vi "myBuriedIntelligence.vi"() -> ()   [LabVIEW 2016]
panel:
  in  "Tab Control":enum32{"Page 1"}(tab)
  out "Array 2":bool[][](array[boolean])
  in  "speed":dbl(slide) scale=0.0..10.0
  in  "Stop":bool
  out "Chosen Path":path
  in  "JPG/JEPG":bool
  in  "Choose Pic Path":path
  out "String":string
  in  "Choose Text Path":path
  out "Read Pic":picture
  out "new picture":picture
  in  "Before Embeded":path
  in  "After Embeded":path
  out "ChosenPath":path
  out "String 2":string
  out "String 3":string
  out "Decoded String":string
  out "Decoded Words Size":i32
  out "Array":bool[][](array[boolean])
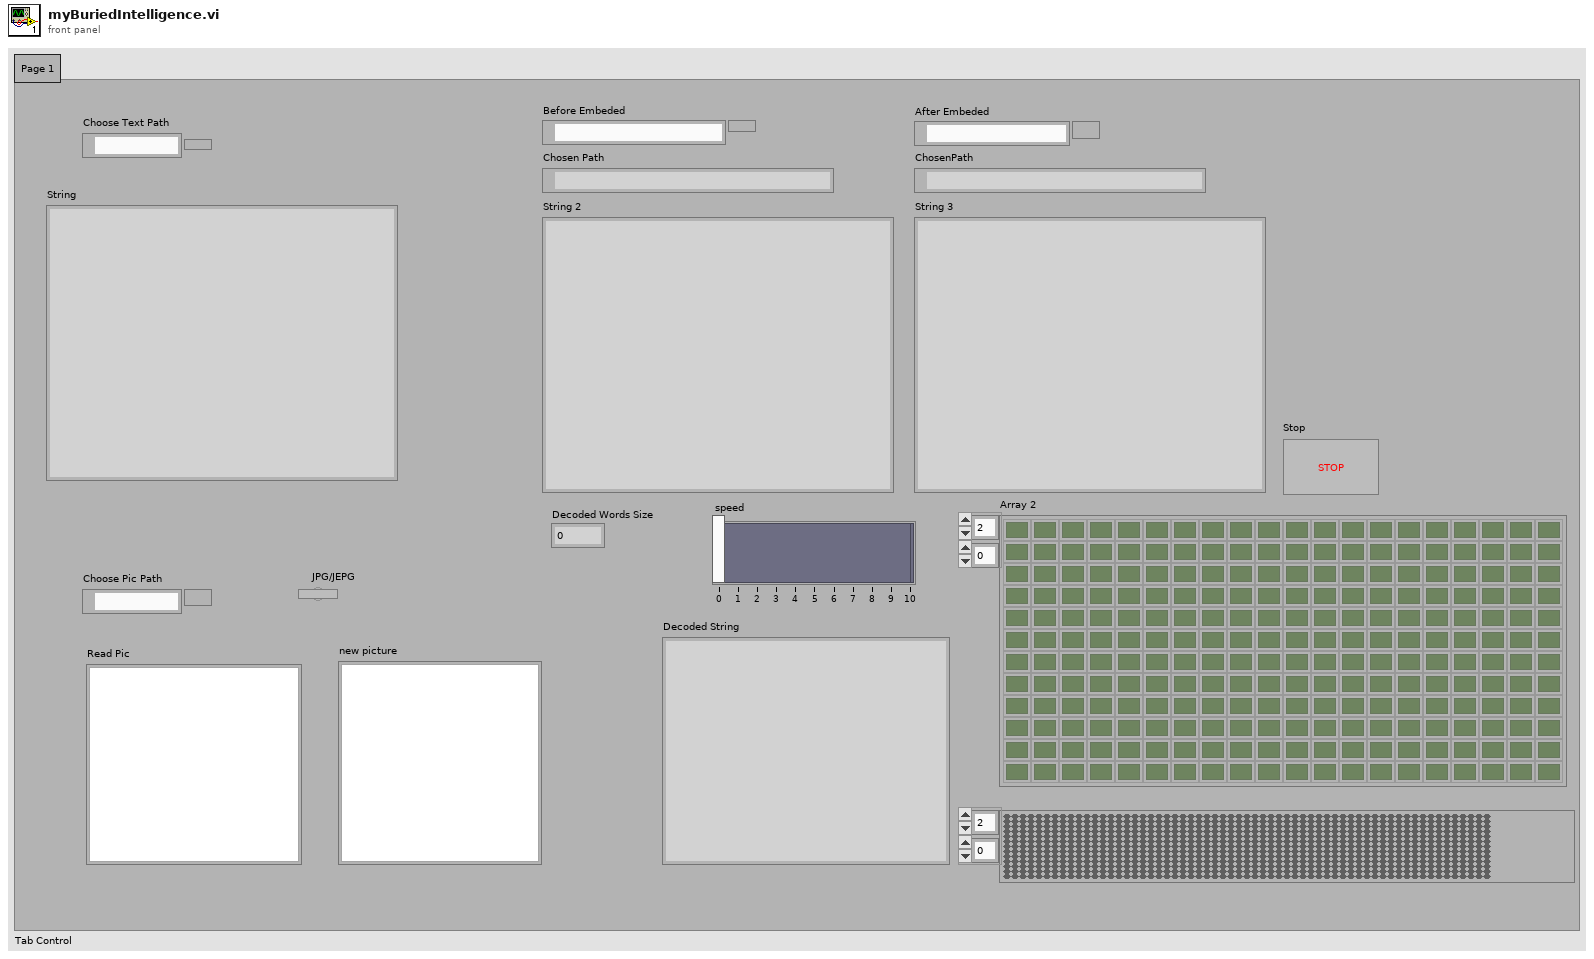
[diagram p1: front panel]
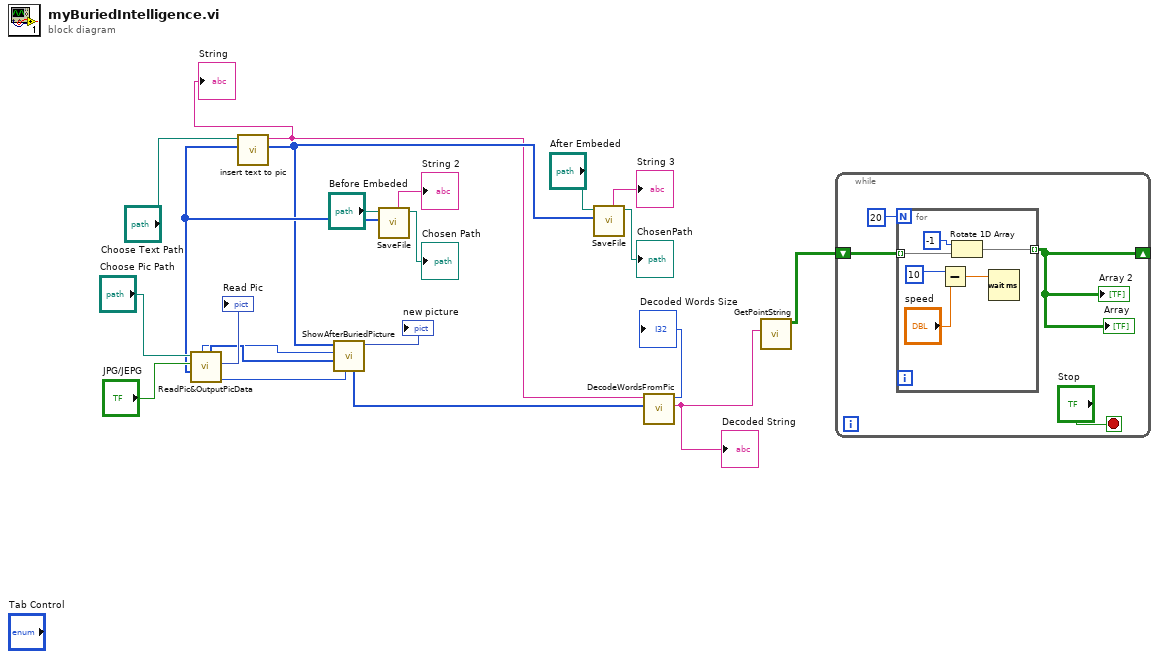
[diagram p0: block diagram]
diagram:
  n1 = call "ReadPic&OutputPicData.vi"("Boolean"="JPG/JEPG", "Path in"="Choose Pic Path") -> ("bottom"=w16:i16, "new picture"=→"Read Pic":picture, "GreenChannel"=w18:u8[], "right"=w17:i16, "RedChannel"=w6:u8[], "BlueChannel"=w14:u8[])  [unwired: 2 in]
  n2 = call "insert text to pic.vi"("BlueChannel in"=w14, "Path"="Choose Text Path") -> ("BlueChannel out(textData)"=w11:u8[], "String"=w4:string)  [unwired: 8 in]
  "String" <- w4
  n3 = call "ShowAfterBuriedPicture.vi"("RedChannel"=w6, "bottom"=w16, "GreenChannel"=w18, "right"=w17, "BlueChannel"=w11) -> ("new picture"=→"new picture":picture, "AfterRecombinedData"=w5:u8[])  [unwired: 5 in]
  n4 = call "SaveFile.vi"("data in"=w14, "File to be opened path"="Before Embeded") -> ("opened path"=→"Chosen Path":path, "String"=→"String 2":string)  [unwired: 8 in]
  n5 = call "SaveFile.vi"("data in"=w11, "File to be opened path"="After Embeded") -> ("opened path"=→"ChosenPath":path, "String"=→"String 3":string)  [unwired: 8 in]
  n6 = call "DecodeWordsFromPic.vi"("AfterRecombinedData"=w5, "String"=w4) -> ("Decoded String"=w2:string, "Decoded Words Size"=→"Decoded Words Size":i32)  [unwired: 8 in]
  "Decoded String" <- w2
  n7 = call "GetPointString.vi"("Decoded String"=w2) -> ("Array"=w1:bool[][])  [unwired: 7 in]
  n8 = while {
    shift-right: [w23] -> _
    shift-left: w1 -> [w26]
    stop <- "Stop" stop-if-true
    n9 = for {
      N: 20 -> [_]
      tunnel: [w31] -> w23 mode=indexing
      tunnel: w26 -> [w30] mode=indexing
      n10 = Subtract(x=10, y="speed") -> (x-y=w28:dbl)
      n11 = Rotate 1D Array(1:w30, 2:-1 ("n")) -> (0:w31:bool[])
      n12 = Wait (ms)(milliseconds to wait=w28) -> ()  [unwired: 1 out]
    }
    "Array" <- w23
    "Array 2" <- w23
  }
